vi "Update DemoService.vi"(8 "error in (no error)":errorcluster, 10 "DemoService":i32, 11 "DIMDemoClient in":refnum<class "DIMDemoClient.lvclass">) -> (0 "error out":errorcluster, 3 "DIMDemoClient out":refnum<class "DIMDemoClient.lvclass">)   [LabVIEW 2012, in "DimActorDemo.lvlib" / "DIMDemoClient.lvclass"]
doc: "Update GUI element DemoService using event."
uses:
  DIMDemoClient.lvclass
  DIMDemoClient.lvclass/DIMDemoClient.ctl
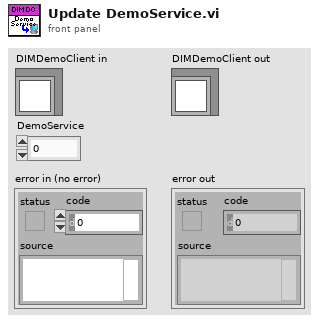
[diagram p1: front panel]
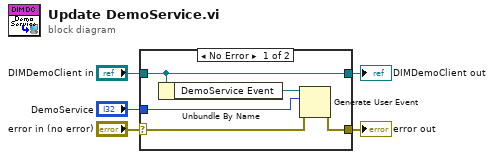
[diagram p0: block diagram]
diagram:
  n1 = case shown="No Error" "error in (no error)" {
    selector: "error in (no error)" -> [w7 w12]
    tunnel: [w6 w12] -> w4
    tunnel: [w10 w11] -> w2
    tunnel: "DIMDemoClient in" -> [w10 w11]
    tunnel: "DemoService" -> [w8 _]
    frame No Error {
      n2 = Unbundle By Name(w10) -> ("DemoService Event"=w9:refnum<user-event>)
      n3 = Generate User Event(user event=w9, event data cluster=w8, error in=w7) -> (error out=w6:errorcluster)  [unwired: 1 out]
    }
    frame Error {
    }
  }
  "error out" <- w4
  "DIMDemoClient out" <- w2
